vi "Find Relative Item.vi"(8 "error in (no error)":errorcluster, 10 "Item Path":string, 11 "Root Item In":refnum<vi>) -> (0 "error out":errorcluster, 2 "Item Ref":refnum<vi>, 3 "Root Item":refnum<vi>)   [LabVIEW 2020, in "Negentropic IDE.lvlib"]
uses:
  Negentropic IDE.lvlib
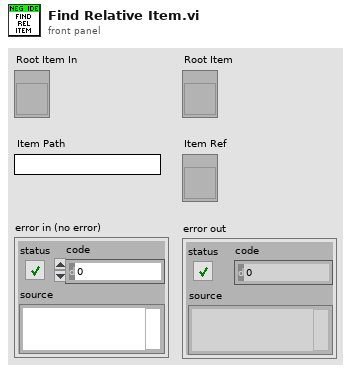
[diagram p1: front panel]
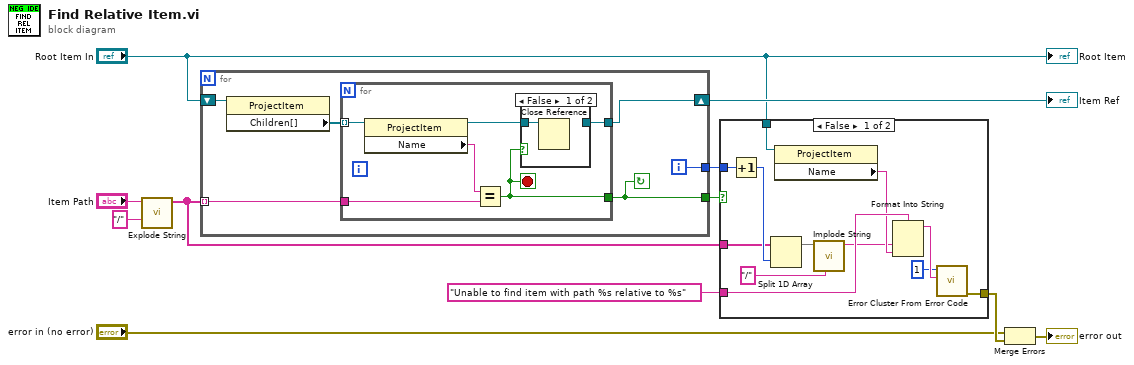
[diagram p0: block diagram]
diagram:
  n1 = call "Explode String.vi"("Delimiter (,)"="/" ("delimiter"), "String"="Item Path") -> ("Array"=w2:string[])  [unwired: 9 in]
  n2 = for {
    tunnel: w2 -> [w17] mode=indexing
    shift-right: [w14] -> w10
    shift-left: "Root Item In" -> [w16]
    tunnel: [w15] -> w11
    tunnel: [w12] -> w9
    i -> [w15]
    stop <- w12 continue-if-true
    n3 = property class="ProjectItem"(reference=w16) -> ("Children[]"=w13:refnum<vi>[])  [unwired: 1 in, 2 out]
    n4 = for {
      tunnel: w17 -> [w22]
      tunnel: [w20] -> w12
      tunnel: [w18] -> w14
      tunnel: w13 -> [w21] mode=indexing
      stop <- w20 stop-if-true
      n5 = property class="ProjectItem"(reference=w21) -> (reference out=w19:refnum<vi>, "Name"=w23:string)  [unwired: 1 in, 1 out]
      n6 = Equal?(x=w23, y=w22) -> (x = y?=w20:bool)
      n7 = case shown="False" w20 {
        tunnel: w19 -> [w24 w25]
        tunnel: [_ w25] -> w18
        frame False {
          n8 = Close Reference(reference=w24) -> ()  [unwired: 1 in, 1 out]
        }
        frame True {
        }
      }
    }
  }
  "Item Ref" <- w10
  n9 = case shown="False" w9 {
    tunnel: w11 -> [w37 _]
    tunnel: w2 -> [w35 _]
    tunnel: "Unable to find item with path %s relative to %s" -> [w34 _]
    tunnel: "Root Item In" -> [w32 _]
    tunnel: [w29 _] -> w6
    frame False {
      n10 = Increment(x=w37) -> (x+1=w36:i32)
      n11 = Split 1D Array(array=w35, index=w36) -> (first subarray=w28:string[])  [unwired: 1 out]
      n12 = property class="ProjectItem"(reference=w32) -> ("Name"=w33:string)  [unwired: 1 in, 2 out]
      n13 = call "Implode String.vi"("Delimiter (,)"="/" ("delimiter"), "Array"=w28) -> ("String"=w26:string)  [unwired: 9 in]
      n14 = Format Into String(format string=w34, w26, w33) -> (resulting string=w31:string)  [unwired: 2 in, 1 out]
      n15 = call <vilib>:"Error Cluster From Error Code.vi"("error message (\"\")"=w31, "error code (0)"=1) -> ("error out"=w29:errorcluster)  [unwired: 7 in]
    }
    frame True {
    }
  }
  n16 = Merge Errors("error in (no error)", w6) -> (→"error out":errorcluster)
  "Root Item" <- "Root Item In"
